vi "Configure Standard Waveform.vi"(0 "RedPitaya connection in":refnum<k5>, 1 "Amplitude (V)":dbl=1.1 min=-1.0 max=1.1, 2 "Frequency":i32=50000000 min=-1 max=50000000, 3 "DC Offset":dbl=1.1 min=-1.0 max=1.1, 4 "Phase":i32=361 min=-360 max=361, 5 "error in":errorcluster, 6 "Channel #":u16(ring)=1 items=["Channel 1"=1, "Channel 2"=2], 7 "Duty Cycle":i32=-1 min=-1 max=100, 8 "Waveform Function":u16(ring) items=["", "Sine", "Square", "Triangle", "Sawtooth UP", "Sawtooth Down", "PWM"], 12 "timeout ms (2000)":i32=2000) -> (14 "RedPitaya connection out":refnum<k5>, 19 "error out":errorcluster)   [LabVIEW 2010, in "RedPitaya.lvlib"]
doc: "Selects the waveform shape, frequency, amplitude, offset, and phase for a standard waveform.\n\nDuty cycle is used only when the shape is set to PWM."
uses:
  RedPitaya.lvlib
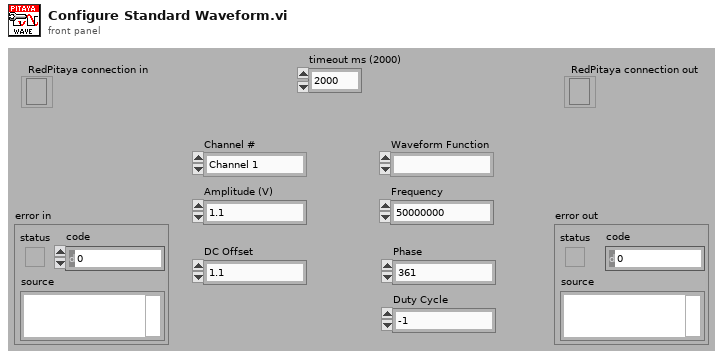
[diagram p1: front panel]
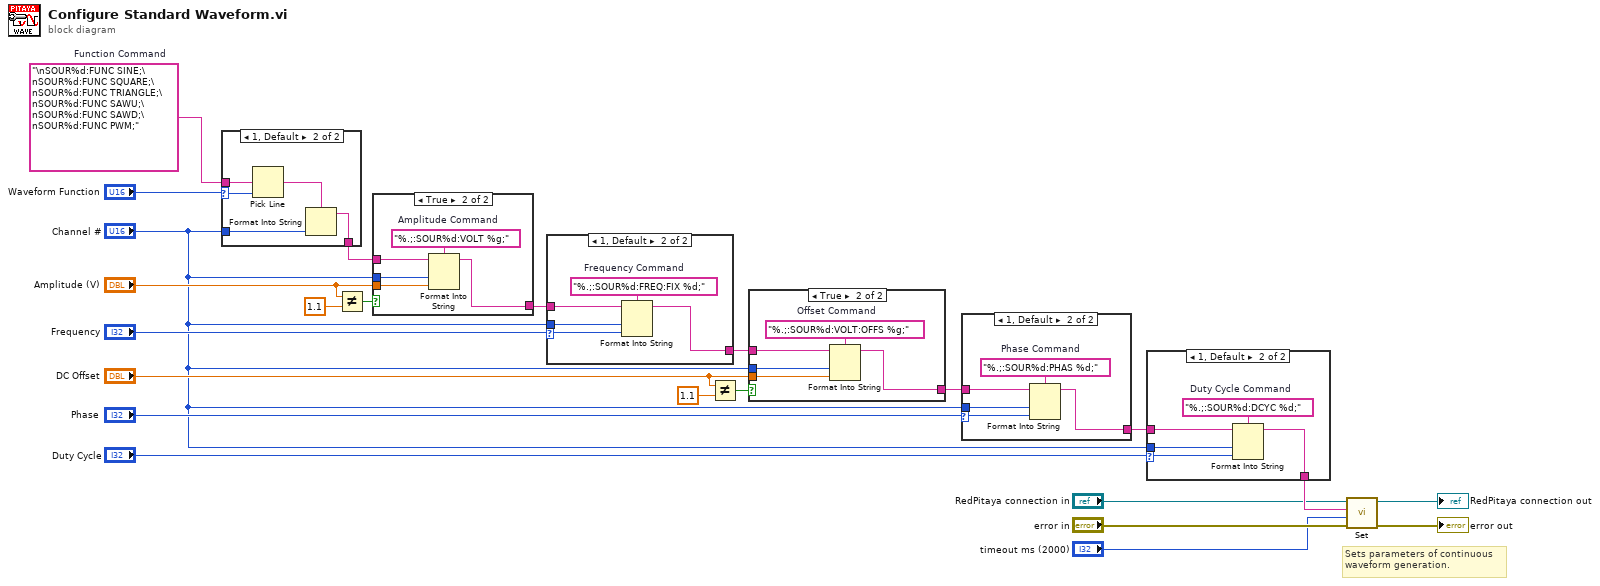
[diagram p0: block diagram]
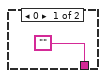
[diagram p7: hidden frame]
diagram:
  w23 = "\nSOUR%d:FUNC SINE;\nSOUR%d:FUNC SQUARE;\nSOUR%d:FUNC TRIANGLE;\nSOUR%d:FUNC SAWU;\nSOUR%d:FUNC SAWD;\nSOUR%d:FUNC PWM;"  # Function Command
  # "Sets parameters of continuous\nwaveform generation."
  n1 = case shown="1, Default" "Waveform Function" {
    selector: "Waveform Function" -> [_ w25]
    tunnel: w23 -> [_ w29]
    tunnel: "Channel #" -> [_ w27]
    tunnel: ["" w26] -> w18
    frame 0 {
    }
    frame 1, Default {
      n2 = Pick Line(multi-line string=w29, line index=w25) -> (output string=w28:string)  [unwired: 1 in]
      n3 = Format Into String(format string=w28, w27) -> (resulting string=w26:string)  [unwired: 2 in, 1 out]
    }
  }
  n4 = Not Equal?(x="Amplitude (V)", y=1.1) -> (x != y?=w11:bool)
  n5 = case shown="True" w11 {
    tunnel: [w30 w35] -> w21
    tunnel: "Amplitude (V)" -> [_ w33]
    tunnel: "Channel #" -> [_ w32]
    tunnel: w18 -> [w30 w31]
    frame False {
    }
    frame True {
      w34 = "%.;:SOUR%d:VOLT %g;"  # Amplitude Command
      n6 = Format Into String(format string=w34, initial string=w31, w32, w33) -> (resulting string=w35:string)  [unwired: 1 in, 1 out]
    }
  }
  n7 = case shown="1, Default" "Frequency" {
    selector: "Frequency" -> [_ w37]
    tunnel: [w36 w41] -> w22
    tunnel: w21 -> [w36 w40]
    tunnel: "Channel #" -> [_ w38]
    frame -1 {
    }
    frame 1, Default {
      w39 = "%.;:SOUR%d:FREQ:FIX %d;"  # Frequency Command
      n8 = Format Into String(format string=w39, initial string=w40, w38, w37) -> (resulting string=w41:string)  [unwired: 1 in, 1 out]
    }
  }
  n9 = Not Equal?(x="DC Offset", y=1.1) -> (x != y?=w6:bool)
  n10 = case shown="True" w6 {
    tunnel: w22 -> [w42 w46]
    tunnel: "DC Offset" -> [_ w45]
    tunnel: [w42 w44] -> w20
    tunnel: "Channel #" -> [_ w43]
    frame False {
    }
    frame True {
      w47 = "%.;:SOUR%d:VOLT:OFFS %g;"  # Offset Command
      n11 = Format Into String(format string=w47, initial string=w46, w43, w45) -> (resulting string=w44:string)  [unwired: 1 in, 1 out]
    }
  }
  n12 = case shown="1, Default" "Phase" {
    selector: "Phase" -> [_ w49]
    tunnel: w20 -> [w48 w52]
    tunnel: [w48 w51] -> w19
    tunnel: "Channel #" -> [_ w50]
    frame 361 {
    }
    frame 1, Default {
      w53 = "%.;:SOUR%d:PHAS %d;"  # Phase Command
      n13 = Format Into String(format string=w53, initial string=w52, w50, w49) -> (resulting string=w51:string)  [unwired: 1 in, 1 out]
    }
  }
  n14 = case shown="1, Default" "Duty Cycle" {
    selector: "Duty Cycle" -> [_ w55]
    tunnel: w19 -> [w54 w58]
    tunnel: "Channel #" -> [_ w57]
    tunnel: [w54 w56] -> w17
    frame -1 {
    }
    frame 1, Default {
      w59 = "%.;:SOUR%d:DCYC %d;"  # Duty Cycle Command
      n15 = Format Into String(format string=w59, initial string=w58, w57, w55) -> (resulting string=w56:string)  [unwired: 1 in, 1 out]
    }
  }
  n16 = call "Set.vi"("error in"="error in", "timeout ms (2000)"="timeout ms (2000)", "SCPI Message"=w17, "RedPitaya connection in"="RedPitaya connection in") -> ("error out"=→"error out":errorcluster, "RedPitaya connection out"=→"RedPitaya connection out":refnum<k5>)  [unwired: 5 in, 1 out]
